vi "global.vi"() -> ()   [LabVIEW 2024]
panel:
  in  "Sample name":string="Elsa"
  in  "Main file path (dialog if empty)":path=path "C:/Users/gyue/Box Sync/Guang Yue/data"
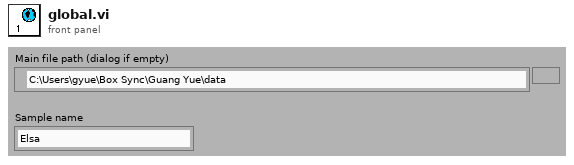
[diagram p1: front panel]
diagram:
